vi "Handle Rectifer Step Selection.vi"(9 "Coords":T1, 10 "Button":u16, 11 "MulticolumnListbox in":refnum<vi>) -> (3 "Row":i32)   [LabVIEW 2019]
uses:
  <vilib>/Utility/miscctls.llb/LVPoint32TypeDef.ctl
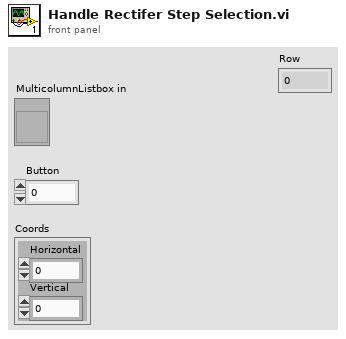
[diagram p1: front panel]
types:
  T1 = typedef "LVPoint32TypeDef.ctl" = cluster{"Horizontal":i32, "Vertical":i32}
  T2 = typedef "LVRowAndColumnTypeDef.ctl" = cluster{"Row":i32, "Column":i32}
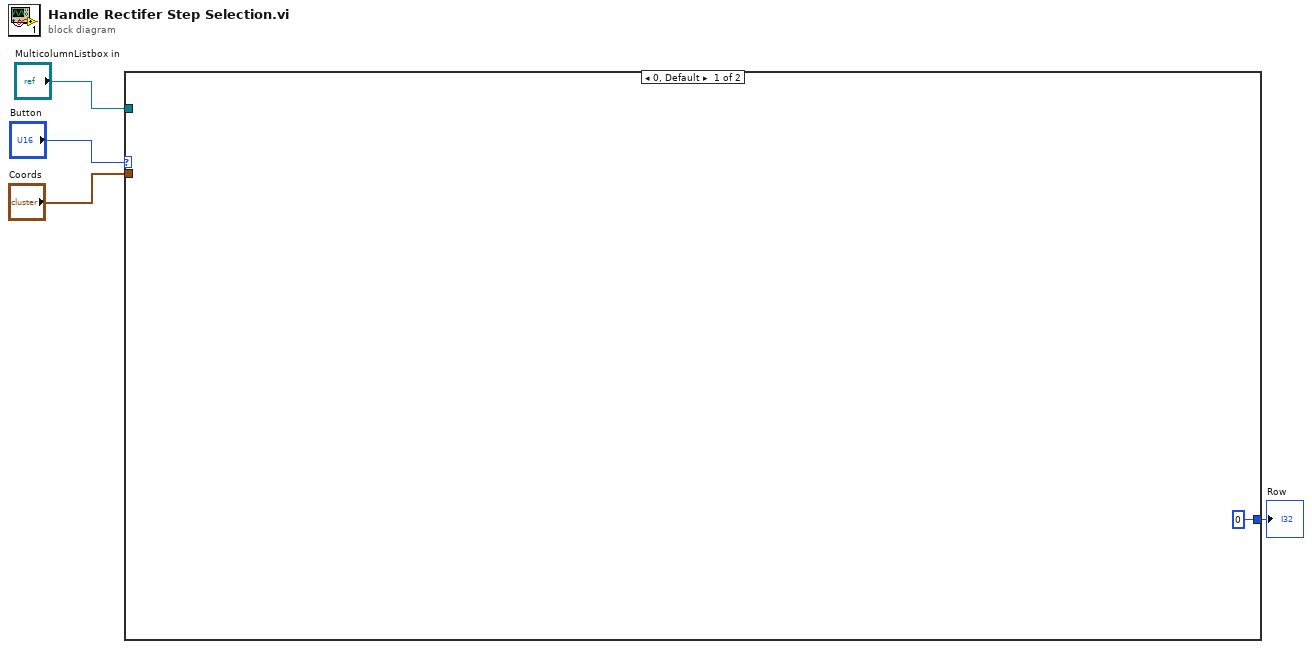
[diagram p0: block diagram]
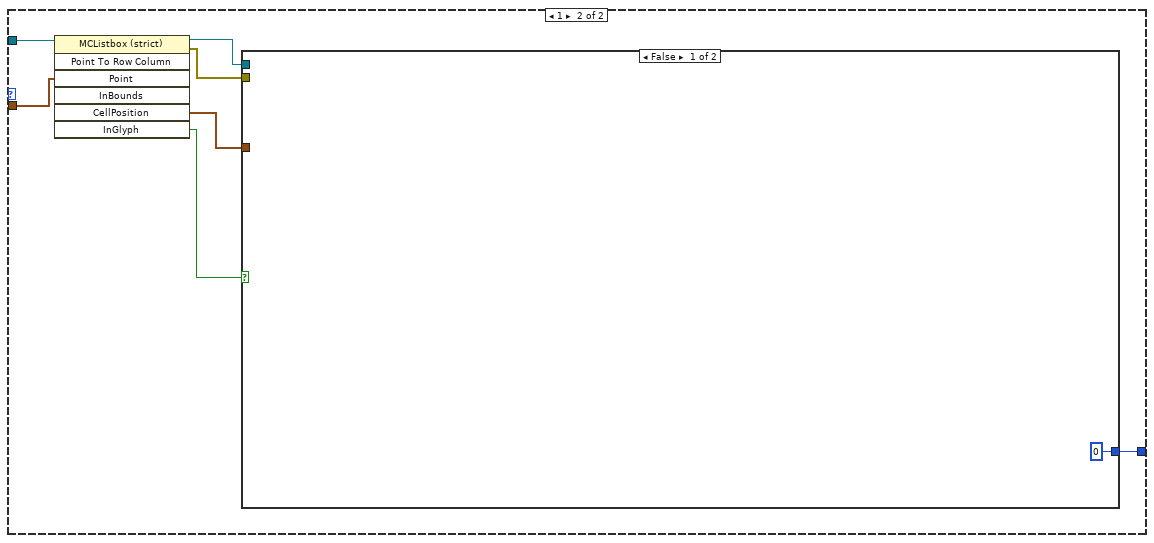
[diagram p2: hidden frame]
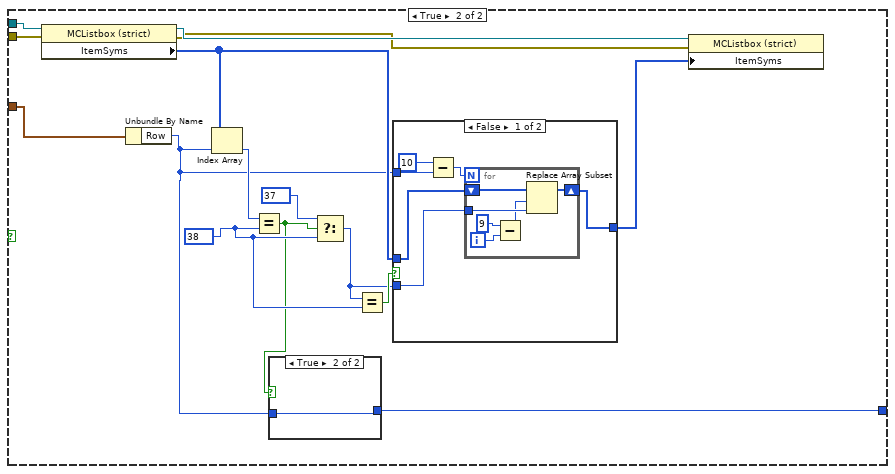
[diagram p3: hidden frame]
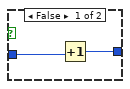
[diagram p4: hidden frame]
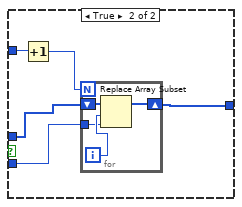
[diagram p5: hidden frame]
diagram:
  n1 = case shown="0, Default" "Button" {
    tunnel: "MulticolumnListbox in" -> [_ w12]
    tunnel: "Coords" -> [_ w9]
    tunnel: [0 ("Row") w6] -> w1
    frame 0, Default {
    }
    frame 1 {
      n2 = invoke class="MCListbox (strict)" method="Point To Row Column"(reference=w12, "Point"=w9) -> (reference out=w8:refnum<vi>, error out=w7:errorcluster, "CellPosition"=w10:T2, "InGlyph"=w11:bool)  [unwired: 5 in, 3 out]
      n3 = case shown="False" w11 {
        tunnel: w10 -> [_ w27]
        tunnel: w8 -> [_ w28]
        tunnel: w7 -> [_ w26]
        tunnel: [0 ("Row") w14] -> w6
        frame False {
        }
        frame True {
          w23 = 38
          n4 = property class="MCListbox (strict)"(reference=w28, error in=w26) -> (reference out=w19:refnum<vi>, error out=w18:errorcluster, "ItemSyms"=w20:i32[])
          n5 = Unbundle By Name(w27) -> ("Row"=w15:i32)
          n6 = Index Array(array=w20, index=w15) -> (element=w25:i32)
          n7 = Equal?(x=w25, y=w23) -> (x = y?=w16:bool)
          n8 = case shown="True" w16 {
            tunnel: w15 -> [w30 w31]
            tunnel: [w29 w31] -> w14
            frame False {
              n9 = Increment(x=w30) -> (x+1=w29:i32)
            }
            frame True {
            }
          }
          n10 = Select(t=37, s=w16, f=w23) -> (s? t:f=w21:i32)
          n11 = Equal?(x=w21, y=w23) -> (x = y?=w22:bool)
          n12 = case shown="False" w22 {
            tunnel: w20 -> [w35 w48]
            tunnel: w21 -> [w32 w47]
            tunnel: [w34 w46] -> w17
            tunnel: w15 -> [w37 w45]
            frame False {
              n13 = Subtract(x=10, y=w37) -> (x-y=w33:i32)
              n14 = for {
                N: w33 -> [_]
                tunnel: w32 -> [w42]
                shift-right: [w41] -> w34
                shift-left: w35 -> [w43]
                i -> [w40]
                n15 = Subtract(x=9, y=w40) -> (x-y=w38:i32)
                n16 = Replace Array Subset(array=w43, new element=w42, index=w38) -> (w41:i32[])
              }
            }
            frame True {
              n17 = Increment(x=w45) -> (x+1=w44:i32)
              n18 = for {
                N: w44 -> [_]
                tunnel: w47 -> [w50]
                shift-right: [w49] -> w46
                shift-left: w48 -> [w52]
                i -> [w51]
                n19 = Replace Array Subset(array=w52, new element=w50, index=w51) -> (w49:i32[])
              }
            }
          }
          n20 = property class="MCListbox (strict)"(reference=w19, error in=w18, "ItemSyms"=w17) -> ()  [unwired: 2 out]
        }
      }
    }
  }
  "Row" <- w1
